vi "sweep_gate_read_lockin.vi"() -> ()   [LabVIEW 2024]
uses:
  <vilib>/Analysis/1siggen.llb/Ramp Pattern by Delta.vi
  <vilib>/Utility/file.llb/Write Delimited Spreadsheet (string).vi
  <vilib>/Utility/file.llb/Write Delimited Spreadsheet (DBL).vi
  C:/Users/Public/OneDrive/Desktop/Keithley_2450_2470_1_4_0_LV2015_NewReadme2_2450-LV2015-1.4.0/Keithley 2450/Keithley 2450.lvlib
  <vilib>/Analysis/NI_AALBase.lvlib
panel:
  in  "Wait for Current Meas":u32=100
  in  "Number of Current Meas":u32=100
  out "Actual voltage":dbl
  in  "Loop?":bool=TRUE
  out "Current set voltage":dbl
  in  "V stepsize":dbl
  in  "start V":dbl
  in  "End V":dbl
  in  "Wait for lock in meas (ms)":i32=2000
  in  "File Path":path=path "C:/Users/Public/OneDrive/Desktop/test.txt"
  out "错误输出":errorcluster
  out "Channel AWaveform Chart":dbl[](graph)
  in  "Channel A Waveform Display":string(combo)="A-R"
  in  "Channel B Waveform Display":string(combo)="Channel_B_Rh1"
  out "Channel B Waveform Chart":dbl[](graph)
  out "AUX-ADC4 (V)":sgl format="%.3f"
  out "AUX-ADC3 (V)":sgl format="%.3f"
  out "AUX-ADC1 (V)":sgl format="%.3f"
  out "AUX-ADC2 (V)":sgl format="%.3f"
  out "R":sgl caption="R (Vrms)" format="%.3p"
  out "X":sgl caption="X (Vrms)" format="%.3p"
  out "Y":sgl caption="Y (Vrms)" format="%.3p"
  out "θ (°)":sgl caption="θ (deg)" format="%.2f"
  out "频率 (Hz)":sgl caption="Freq (Hz)" format="%#.3f"
  out "噪声":sgl caption="Noise(Vrms)" format="%.3p"
  out "Rh1":sgl caption="Rh1 (Vrms)" format="%.3p"
  out "θh1 (°)":sgl caption="θh1 (deg)" format="%.2f"
  out "Xh1":sgl caption="Xh1 (Vrms)" format="%.3p"
  out "Yh1":sgl caption="Yh1 (Vrms)" format="%.3p"
  out "X 2":sgl caption="X (Vrms)" format="%.3p"
  out "Y 2":sgl caption="Y (Vrms)" format="%.3p"
  out "R 2":sgl caption="R (Vrms)" format="%.3p"
  out "θ (°) 2":sgl caption="θ (deg)" format="%.2f"
  out "频率 (Hz) 2":sgl caption="Freq (Hz)" format="%#.3f"
  out "噪声 2":sgl caption="Noise(Vrms)" format="%.3p"
  out "Xh1 2":sgl caption="Xh1 (Vrms)" format="%.3p"
  out "Yh1 2":sgl caption="Yh1 (Vrms)" format="%.3p"
  out "Rh1 2":sgl caption="Rh1 (Vrms)" format="%.3p"
  out "θh1 (°) 2":sgl caption="θh1 (deg)" format="%.2f"
  in  "A Sensitivity":u16(ring)=20 items=["1 nV/fA", "2 nV/fA", "5 nV/fA", "10 nV/fA", "20 nV/fA", "50 nV/fA", "100 nV/fA", "200 nV/fA", "500 nV/fA", "1 uV/pA", "2 uV/pA", "5 uV/pA", "10 uV/pA", "20 uV/pA", "50 uV/pA", "100 uV/pA", "200 uV/pA", "500 uV/pA", "1 mV/nA", "2 mV/nA", "5 mV/nA", "10 mV/nA", "20 mV/nA", "50 mV/nA", "100 mV/nA", "200 mV/nA", "500 mV/nA", "1 V/uA"]
  in  "B Sensitivity":u16(ring)=17 items=["1 nV/fA", "2 nV/fA", "5 nV/fA", "10 nV/fA", "20 nV/fA", "50 nV/fA", "100 nV/fA", "200 nV/fA", "500 nV/fA", "1 uV/pA", "2 uV/pA", "5 uV/pA", "10 uV/pA", "20 uV/pA", "50 uV/pA", "100 uV/pA", "200 uV/pA", "500 uV/pA", "1 mV/nA", "2 mV/nA", "5 mV/nA", "10 mV/nA", "20 mV/nA", "50 mV/nA", "100 mV/nA", "200 mV/nA", "500 mV/nA", "1 V/uA"]
  out "序列号":string
  in  "Num Lock in Points":i32=100
  in  "OE1022D":refnum<visa-resource-name>="COM6"
  in  "Limit Reached 2":bool
  in  "Current Compliance Limit (0.1)":dbl=5e-08
  in  "Time between Current Meas (ms)":u32=100
  out "Current":dbl caption="Measured Current (A)"
  out "XY Graph":cluster{dbl[], dbl[]}(graph)
  out "error out":errorcluster
  in  "error in (no error)":errorcluster
  in  "VISA resource name 2":refnum<visa-resource-name>="GPIB0::18::INSTR"
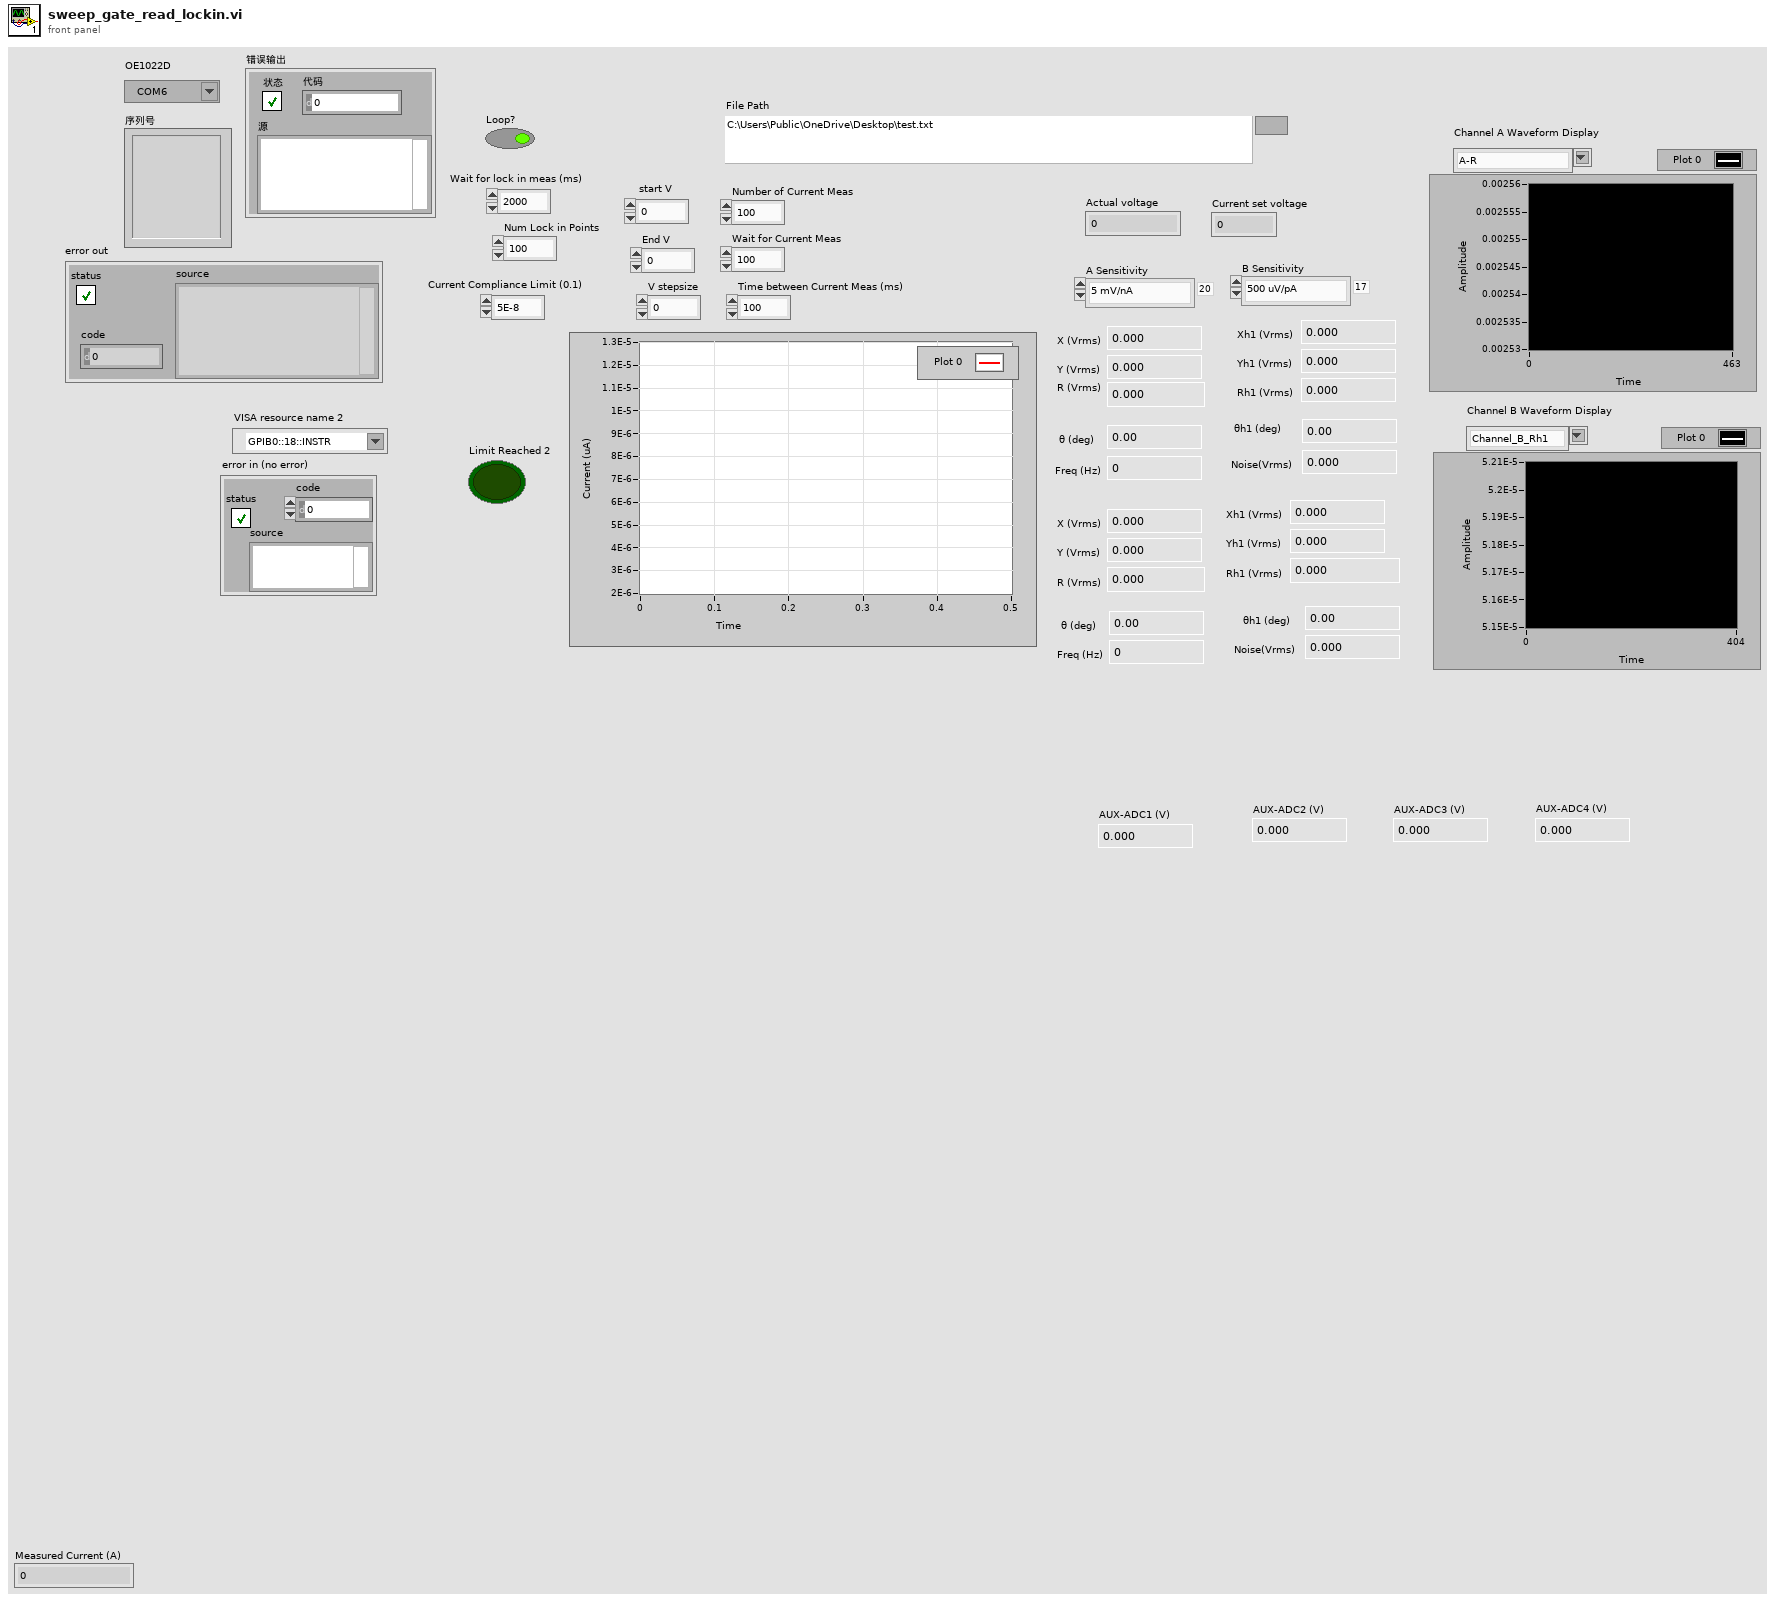
[diagram p1: front panel]
types:
  T1 = cluster{"AD1":dbl[], "AD2":dbl[], "AD3":dbl[], "AD4":dbl[]}
  T2 = cluster{"XB":dbl[], "YB":dbl[], "FrequencyB":dbl[], "NoiseB":dbl[], "Xh1B":dbl[], "Yh1B":dbl[], "Xh2B":dbl[], "Yh2B":dbl[], "Xh2B":dbl[]}
  T3 = cluster{"XA":dbl[], "YA":dbl[], "FrequencyA":dbl[], "NoiseA":dbl[], "Xh1A":dbl[], "Yh1A":dbl[], "Xh2A":dbl[], "Yh2A":dbl[]}
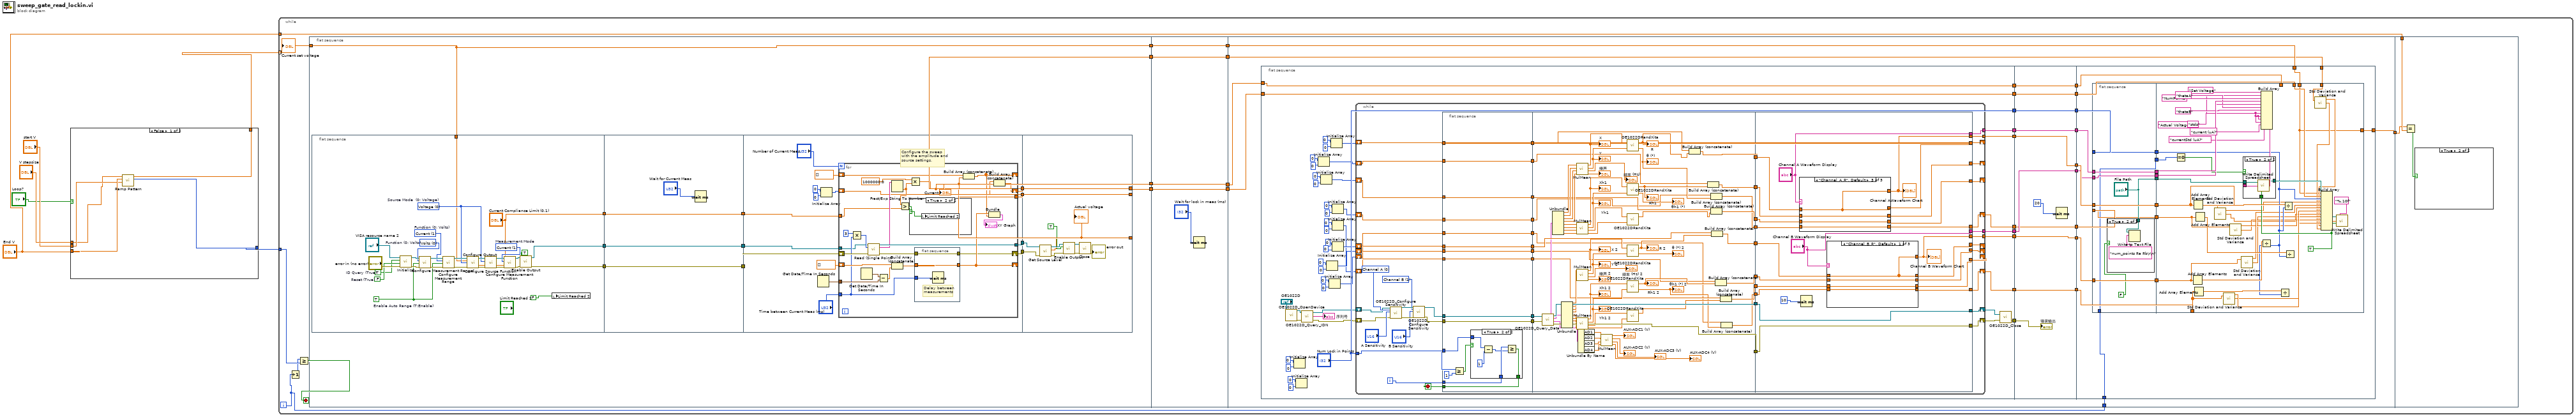
[diagram p0: block diagram]
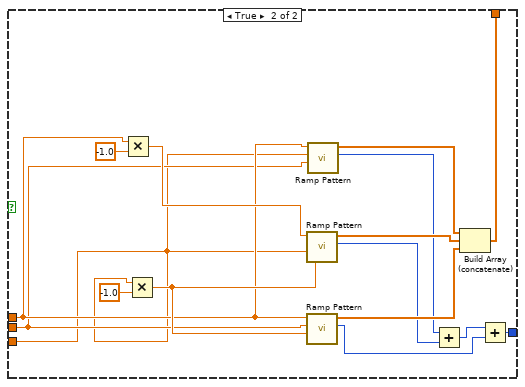
[diagram p2: hidden frame]
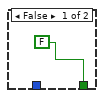
[diagram p4: hidden frame]
diagram:
  n1 = case shown="False" "Loop?" {
    tunnel: [w8 w20] -> w6
    tunnel: [w7 w15] -> w5
    tunnel: "V stepsize" -> [w9 w14]
    tunnel: "start V" -> [w10 w13]
    tunnel: "End V" -> [w11 w12]
    frame False {
      n2 = call-poly <vilib>:"Ramp Pattern.vi"("start"=w10, "end"=w11, "delta"=w9) -> ("samples"=w7:i32, "Ramp Pattern"=w8:dbl[])  [unwired: 6 in, 1 out]
    }
    frame True {
      n3 = Multiply(x=w14, y=-1.0) -> (x*y=w25:dbl)
      n4 = Multiply(x=w12, y=-1.0) -> (x*y=w24:dbl)
      n5 = call-poly <vilib>:"Ramp Pattern.vi"("start"=w12, "end"=w24, "delta"=w25) -> ("samples"=w18:i32, "Ramp Pattern"=w22:dbl[])  [unwired: 6 in, 1 out]
      n6 = call-poly <vilib>:"Ramp Pattern.vi"("start"=w24, "end"=w13, "delta"=w14) -> ("samples"=w17:i32, "Ramp Pattern"=w21:dbl[])  [unwired: 6 in, 1 out]
      n7 = call-poly <vilib>:"Ramp Pattern.vi"("start"=w13, "end"=w12, "delta"=w14) -> ("samples"=w19:i32, "Ramp Pattern"=w23:dbl[])  [unwired: 6 in, 1 out]
      n8 = Add(x=w19, y=w18) -> (x+y=w16:i32)
      n9 = Build Array (concatenate)(w23, w22, w21) -> (w20:dbl[])
      n10 = Add(x=w16, y=w17) -> (x+y=w15:i32)
    }
  }
  n11 = while {
    tunnel: w6 -> [w40] mode=indexing
    tunnel: w5 -> [w42]
    tunnel: "End V" -> [w28]
    i -> [w30]
    stop <- w41 stop-if-true
    n12 = Increment(x=w30) -> (x+1=w39:i32)
    n13 = Greater Or Equal?(x=w39, y=w42) -> (x >= y?=w41:bool)
    n14 = flat-sequence {
      tunnel: w40 -> [w49]
      tunnel: [w56] -> w37
      tunnel: [w49] -> w36
      tunnel: [w50] -> w33
      tunnel: [w55] -> w31
      tunnel: [w146] -> w38
      tunnel: w37 -> [w146]
      tunnel: w36 -> [w145]
      tunnel: [w145] -> w35
      tunnel: [w144] -> w34
      tunnel: w33 -> [w144]
      tunnel: [w143] -> w32
      tunnel: w31 -> [w143]
      tunnel: w38 -> [w157]
      tunnel: w35 -> [w154]
      tunnel: w34 -> [w153]
      tunnel: w32 -> [w150]
      tunnel: w30 -> [w149]
      tunnel: [w148] -> w29
      tunnel: w29 -> [w504]
      tunnel: w28 -> [w505]
      frame #0 {
        n15 = flat-sequence {
          tunnel: w49 -> [w60]
          tunnel: [w59] -> w48
          tunnel: ["Current Compliance Limit (0.1)"] -> w46
          tunnel: [w57] -> w44
          tunnel: w48 -> [w87]
          tunnel: [w87] -> w47
          tunnel: w46 -> [w86]
          tunnel: [w86] -> w45
          tunnel: w44 -> [w85]
          tunnel: [w85] -> w43
          tunnel: [w98] -> w54
          tunnel: [w97] -> w53
          tunnel: [w93] -> w52
          tunnel: [w92] -> w51
          tunnel: w47 -> [w90]
          tunnel: w45 -> [w89]
          tunnel: w43 -> [w88]
          tunnel: [w141] -> w55
          tunnel: [w142] -> w56
          tunnel: w54 -> [w134]
          tunnel: w53 -> [w135]
          tunnel: w52 -> [w142]
          tunnel: w51 -> [w141]
          tunnel: [w132] -> w50
          frame #0 {
            w61 = u16 0 items=["Voltage", "Current"]  # Source Mode  (0: Voltage)
            w62 = u16 1 items=["Volts", "Current", "Auto Resistance", "Manual Resistance", "Digitize Voltage", "Digitize Current"]  # Measurement Mode
            w66 = TRUE  # Enable Auto Range (T:Enable)
            w64 = u16 1 items=["Volts", "Current", "Resistance"]  # Function (0: Volts)
            w65 = u16 0 items=["Volts", "Current", "Resistance"]  # Function (0: Volts)
            w68 = FALSE  # Reset (True)
            w67 = TRUE  # ID Query (True)
            n16 = call "Initialize.vi"("error in (no error)"="error in (no error)", "Reset (True)"=w68, "ID Query (True)"=w67, "VISA resource name"="VISA resource name 2") -> ("error out"=w72:errorcluster, "VISA resource name out"=w71:refnum<visa-resource-name>)  [unwired: 6 in]
            n17 = call "Configure Measurement Range.vi"("error in (no error)"=w72, "Enable Auto Range (T:Enable)"=w66, "Function (0: Volts)"=w65, "VISA resource name"=w71) -> ("error out"=w70:errorcluster, "VISA resource name out"=w69:refnum<visa-resource-name>)  [unwired: 6 in]
            n18 = call "Configure Measurement Range.vi"("error in (no error)"=w70, "Enable Auto Range (T:Enable)"=w66, "Function (0: Volts)"=w64, "VISA resource name"=w69) -> ("error out"=w80:errorcluster, "VISA resource name out"=w81:refnum<visa-resource-name>)  [unwired: 6 in]
            n19 = call "Configure Output.vi"("VISA resource name"=w81, "Source Level (0)"=w60, "Source Mode  (0: Voltage)"=w61, "Source Limit Level (0.1)"="Current Compliance Limit (0.1)", "error in (no error)"=w80) -> ("VISA resource name out"=w73:refnum<visa-resource-name>, "error out"=w74:errorcluster)  [unwired: 9 in]
            n20 = call "Configure Source Function.vi"("error in (no error)"=w74, "Function (0: Volts)"=w61, "VISA resource name"=w73) -> ("error out"=w76:errorcluster, "VISA resource name out"=w77:refnum<visa-resource-name>)  [unwired: 7 in]
            n21 = call "Configure Measurement Function.vi"("error in (no error)"=w76, "Function (0: Volts)"=w62, "VISA resource name"=w77) -> ("error out"=w78:errorcluster, "VISA resource name out"=w79:refnum<visa-resource-name>)  [unwired: 7 in]
            n22 = call "Enable Output.vi"("error in (no error)"=w78, "Enable Output (T: Enable)"=TRUE, "VISA resource name"=w79) -> ("error out"=w57:errorcluster, "VISA resource name out"=w59:refnum<visa-resource-name>)  [unwired: 7 in]
            n23 = local write "Limit Reached 2"(FALSE) -> ()
          }
          frame #1 {
            n24 = Wait (ms)(milliseconds to wait="Wait for Current Meas") -> ()  [unwired: 1 out]
          }
          frame #2 {
            # "Configure the sweep with the amplitude and source settings."
            n25 = Get Date/Time In Seconds() -> (seconds since 1Jan1904=w102:timestamp)
            n26 = Initialize Array(0, 0) -> (w94:i32[])
            n27 = for {
              N: "Number of Current Meas" -> [_]
              shift-right: [w116] -> w97
              shift-left: w88 -> [w118]
              tunnel: w102 -> [w126]
              shift-right: [w122] -> _
              shift-left: dbl[] [] -> [w125]
              shift-right: [w121] -> _
              shift-left: dbl[] [] -> [w124]
              tunnel: "Time between Current Meas (ms)" -> [w114]
              tunnel: [w112] -> w98
              tunnel: w89 -> [w110]
              tunnel: [w106] -> w93
              shift-right: [w108] -> w92
              shift-left: w94 -> [w107]
              tunnel: w90 -> [w104]
              n28 = Multiply(x=u32 3, y=w114) -> (x*y=w115:u32)
              n29 = Get Date/Time In Seconds() -> (seconds since 1Jan1904=w127:timestamp)
              n30 = call "Read (Single Point).vi"("VISA resource name"=w104, "Timeout (10000 ms)"=w115, "error in (no error)"=w118) -> ("VISA resource name out"=w112:refnum<visa-resource-name>, "Data out"=w111:string, "error out"=w117:errorcluster)  [unwired: 10 in]
              n31 = Subtract(x=w127, y=w126) -> (x-y=w119:dbl)
              n32 = Fract/Exp String To Number(string=w111) -> (number=w103:dbl)  [unwired: 3 in, 1 out]
              n33 = Build Array (concatenate)(w125, w119) -> (w123:dbl[])
              n34 = Greater?(x=w103, y=w110) -> (0:w109:bool)
              n35 = case shown="True" w109 {
                selector: w109 -> [_ w128]
                frame False {
                }
                frame True {
                  n36 = local write "Limit Reached 2"(w128) -> ()
                }
              }
              n37 = Multiply(x=1000000.0, y=w103) -> (x*y=w106:dbl)
              "Current" <- w106
              n38 = flat-sequence {
                tunnel: w123 -> [w131]
                tunnel: [w131] -> w122
                tunnel: w114 -> [w130]
                tunnel: w117 -> [w129]
                tunnel: [w129] -> w116
                frame #0 {
                  # "Delay between\nmeasurements"
                  n39 = Wait (ms)(milliseconds to wait=w130) -> ()  [unwired: 1 out]
                }
              }
              n40 = Build Array (concatenate)(w124, w106) -> (w121:dbl[])
              n41 = Bundle(w122, w121) -> (→"XY Graph":cluster{dbl[], dbl[]})  [unwired: 1 in]
              n42 = Build Array (concatenate)(w107, w106) -> (w108:dbl[])
            }
          }
          frame #3 {
            n43 = call "Get Source Level.vi"("error in (no error)"=w135, "VISA resource name"=w134) -> ("error out"=w139:errorcluster, "Voltage Level Out"=w132:dbl, "VISA resource name out"=w140:refnum<visa-resource-name>)  [unwired: 6 in, 1 out]
            "Actual voltage" <- w132
            n44 = call "Enable Output.vi"("error in (no error)"=w139, "Enable Output (T: Enable)"=TRUE, "VISA resource name"=w140) -> ("error out"=w137:errorcluster, "VISA resource name out"=w136:refnum<visa-resource-name>)  [unwired: 7 in]
            n45 = call "Close.vi"("error in (no error)"=w137, "VISA resource name"=w136) -> ("error out"=→"error out":errorcluster)  [unwired: 9 in]
          }
        }
      }
      frame #1 {
        n46 = Wait (ms)(milliseconds to wait="Wait for lock in meas (ms)") -> ()  [unwired: 1 out]
      }
      frame #2 {
        n47 = flat-sequence {
          tunnel: [w195] -> w172
          tunnel: [w194] -> w171
          tunnel: ["Num Lock in Points"] -> w170
          tunnel: [w189] -> w169
          tunnel: [w193] -> w168
          tunnel: [w192] -> w167
          tunnel: [w179] -> w166
          tunnel: [w180] -> w165
          tunnel: w157 -> [w174]
          tunnel: [w174] -> w155
          tunnel: w153 -> [w173]
          tunnel: [w173] -> w151
          tunnel: w172 -> [w425]
          tunnel: [w425] -> w164
          tunnel: w171 -> [w424]
          tunnel: [w424] -> w163
          tunnel: w170 -> [w423]
          tunnel: [w423] -> w162
          tunnel: w169 -> [w421]
          tunnel: [w420] -> w161
          tunnel: w168 -> [w420]
          tunnel: w167 -> [w419]
          tunnel: [w419] -> w160
          tunnel: [w418] -> w159
          tunnel: w166 -> [w418]
          tunnel: w165 -> [w417]
          tunnel: [w417] -> w158
          tunnel: [w416] -> w156
          tunnel: w155 -> [w416]
          tunnel: [w415] -> w152
          tunnel: w151 -> [w415]
          tunnel: w164 -> [w442]
          tunnel: w163 -> [w441]
          tunnel: w162 -> [w440]
          tunnel: w161 -> [w438]
          tunnel: w160 -> [w437]
          tunnel: w159 -> [w435]
          tunnel: w158 -> [w433]
          tunnel: w156 -> [w432]
          tunnel: w154 -> [w431]
          tunnel: w152 -> [w430]
          tunnel: w150 -> [w429]
          tunnel: w149 -> [w427]
          tunnel: [w426] -> w148
          frame #0 {
            n48 = call "OE1022D_OpenDevice.vi"("VISA resource name"="OE1022D") -> ("VISA资源名称输出"=w217:refnum<visa-resource-name>, "错误输出"=w216:errorcluster)  [unwired: 17 in]
            n49 = Initialize Array(0, 0) -> ()  [unwired: 1 out]
            n50 = Initialize Array(0, 0) -> ()  [unwired: 1 out]
            n51 = call "OE1022D_Query_IDN.vi"("错误输入（无错误）"=w216, "VISA resource name"=w217) -> ("错误输出"=w187:errorcluster, "序列号"=→"序列号":string, "VISA resource name out"=w188:refnum<visa-resource-name>)  [unwired: 1 in]
            n52 = Initialize Array(0, 0) -> (w202:i32[])
            n53 = Initialize Array(0, 0) -> (w203:i32[])
            n54 = Initialize Array(0, 0) -> (w196:i32[])
            n55 = Initialize Array(0, 0) -> (w197:i32[])
            n56 = Initialize Array(0, 0) -> (w213:i32[])
            n57 = Initialize Array(0, 0) -> (w181:i32[])
            n58 = Initialize Array(0, 0) -> (w208:i32[])
            n59 = Initialize Array(0, 0) -> (w182:i32[])
            n60 = while {
              shift-right: [w270] -> _
              shift-left: w213 -> [w269]
              shift-right: [w267] -> _
              shift-left: w208 -> [w266]
              tunnel: "Num Lock in Points" -> [w259]
              shift-right: [w247] -> _
              shift-left: w202 -> [w249]
              shift-right: [w243] -> _
              shift-left: w203 -> [w246]
              shift-right: [w236] -> _
              shift-left: w196 -> [w242]
              shift-right: [w235] -> _
              shift-left: w197 -> [w241]
              tunnel: [w234] -> w195
              tunnel: [w233] -> w194
              tunnel: [w232] -> w193
              tunnel: [w231] -> w192
              shift-right: [w230] -> w191
              shift-left: w187 -> [w227]
              shift-right: [w229] -> w190
              shift-left: w188 -> [w228]
              shift-right: [w219] -> w179
              shift-left: w182 -> [w223]
              shift-right: [w220] -> w180
              shift-left: w181 -> [w221]
              i -> [w261]
              stop <- w260 stop-if-true
              w252 = u8 1 items=["Channel A", "Channel B"] ("OE1022D A/B")
              w258 = u8 0 items=["Channel A", "Channel B"] ("OE1022D A/B")
              n61 = call "OE1022D_Configure Sensitivity.vi"("VISA resource name"=w228, "OE1022D A/B"=w258, "Sensitivity"="A Sensitivity", "error in (no error)"=w227) -> ("VISA resource name out"=w253:refnum<visa-resource-name>, "error out"=w254:errorcluster)  [unwired: 14 in]
              n62 = call "OE1022D_Configure Sensitivity.vi"("VISA resource name"=w253, "OE1022D A/B"=w252, "Sensitivity"="B Sensitivity", "error in (no error)"=w254) -> ("VISA resource name out"=w256:refnum<visa-resource-name>, "error out"=w255:errorcluster)  [unwired: 14 in]
              n63 = flat-sequence {
                tunnel: w266 -> [w285]
                tunnel: w269 -> [w286]
                tunnel: w256 -> [w287]
                tunnel: w255 -> [w288]
                tunnel: [w288] -> w265
                tunnel: [w287] -> w264
                tunnel: [w286] -> w263
                tunnel: [w285] -> w262
                tunnel: w261 -> [w284]
                tunnel: [w283] -> w260
                tunnel: w259 -> [w281]
                tunnel: [w279] -> w250
                tunnel: w249 -> [w279]
                tunnel: w246 -> [w278]
                tunnel: [w278] -> w245
                tunnel: w242 -> [w277]
                tunnel: w241 -> [w276]
                tunnel: [w277] -> w240
                tunnel: [w276] -> w239
                tunnel: [w275] -> w224
                tunnel: w223 -> [w275]
                tunnel: [w274] -> w222
                tunnel: w221 -> [w274]
                tunnel: [w365] -> w273
                tunnel: [w364] -> w272
                tunnel: [w317] -> w271
                tunnel: [w313] -> w268
                tunnel: w265 -> [w367]
                tunnel: w264 -> [w366]
                tunnel: w263 -> [w318]
                tunnel: w262 -> [w315]
                tunnel: w250 -> [w311]
                tunnel: [w310] -> w248
                tunnel: w245 -> [w308]
                tunnel: [w307] -> w244
                tunnel: w240 -> [w303]
                tunnel: w239 -> [w304]
                tunnel: [w302] -> w238
                tunnel: [w301] -> w237
                tunnel: [w297] -> w226
                tunnel: [w299] -> w225
                tunnel: w224 -> [w296]
                tunnel: w222 -> [w295]
                tunnel: w273 -> [w388]
                tunnel: w272 -> [w389]
                tunnel: w271 -> [w387]
                tunnel: [w385] -> w270
                tunnel: w268 -> [w381]
                tunnel: [w380] -> w267
                tunnel: [w389] -> w229
                tunnel: [w388] -> w230
                tunnel: w248 -> [w386]
                tunnel: [w384] -> w247
                tunnel: w244 -> [w383]
                tunnel: [w382] -> w243
                tunnel: w238 -> [w376]
                tunnel: w237 -> [w379]
                tunnel: [w378] -> w236
                tunnel: [w377] -> w235
                tunnel: [w375] -> w234
                tunnel: [w374] -> w233
                tunnel: ["Channel A Waveform Display"] -> w232
                tunnel: ["Channel B Waveform Display"] -> w231
                tunnel: w226 -> [w370]
                tunnel: [w369] -> w219
                tunnel: [w368] -> w220
                tunnel: w225 -> [w371]
                frame #0 {
                  n64 = Greater Or Equal?(x=w281, y=1) -> (x >= y?=w280:bool)
                  n65 = case shown="True" w280 {
                    tunnel: w284 -> [_ w294]
                    tunnel: [FALSE w293] -> w283
                    tunnel: w281 -> [_ w290]
                    frame False {
                    }
                    frame True {
                      n66 = Subtract(x=w290, y=1) -> (x-y=w291:i32)
                      n67 = Greater Or Equal?(x=w294, y=w291) -> (x >= y?=w293:bool)
                    }
                  }
                }
                frame #1 {
                  n68 = call "OE1022D_Query_Data.vi"("错误输入（无错误）"=w367, "VISA resource name"=w366) -> ("error out"=w365:errorcluster, "输出簇ADC"=w321:T1, "输出簇B"=w320:T2, "VISA resource name out"=w364:refnum<visa-resource-name>, "输出簇A"=w314:T3)  [unwired: 3 in]
                  n69 = Unbundle(w314) -> ("XA"=w326:dbl[], "YA"=w327:dbl[], "FrequencyA"=w328:dbl[], "NoiseA"=w329:dbl[], "Xh1A"=w334:dbl[], "Yh1A"=w335:dbl[], "Xh2A"=w336:dbl[], "Yh2A"=w337:dbl[])
                  n70 = Unbundle(w320) -> ("XB"=w350:dbl[], "YB"=w349:dbl[], "FrequencyB"=w348:dbl[], "NoiseB"=w347:dbl[], "Xh1B"=w346:dbl[], "Yh1B"=w345:dbl[], "Xh2B"=w344:dbl[], "Yh2B"=w343:dbl[])  [unwired: 1 out]
                  n71 = call "MulMean.vi"("IN 4"=w329, "IN 3"=w328, "IN 2"=w327, "IN 1"=w326) -> ("mean 4"=→"噪声":dbl, "mean 3"=→"频率 (Hz)":dbl, "mean 2"=w332:dbl, "mean 1"=w331:dbl)  [unwired: 4 in]
                  "X" <- w331
                  "Y" <- w332
                  n72 = call "MulMean.vi"("IN 4"=w337, "IN 3"=w336, "IN 2"=w335, "IN 1"=w334) -> ("mean 4"=w342:dbl, "mean 3"=w341:dbl, "mean 2"=w339:dbl, "mean 1"=w338:dbl)  [unwired: 4 in]
                  "Xh1" <- w338
                  "Yh1" <- w339
                  n73 = call "MulMean.vi"("IN 4"=w347, "IN 3"=w348, "IN 2"=w349, "IN 1"=w350) -> ("mean 4"=→"噪声 2":dbl, "mean 3"=→"频率 (Hz) 2":dbl, "mean 2"=w355:dbl, "mean 1"=w354:dbl)  [unwired: 4 in]
                  "X 2" <- w354
                  "Y 2" <- w355
                  n74 = call "MulMean.vi"("IN 4"=w343, "IN 3"=w344, "IN 2"=w345, "IN 1"=w346) -> ("mean 4"=w359:dbl, "mean 3"=w358:dbl, "mean 2"=w357:dbl, "mean 1"=w356:dbl)  [unwired: 4 in]
                  "Xh1 2" <- w356
                  "Yh1 2" <- w357
                  n75 = Unbundle By Name(w321) -> ("AD1"=w360:dbl[], "AD2"=w361:dbl[], "AD3"=w362:dbl[], "AD4"=w363:dbl[])
                  n76 = call "MulMean.vi"("IN 4"=w363, "IN 3"=w362, "IN 2"=w361, "IN 1"=w360) -> ("mean 4"=→"AUX-ADC4 (V)":dbl, "mean 3"=→"AUX-ADC3 (V)":dbl, "mean 2"=→"AUX-ADC2 (V)":dbl, "mean 1"=→"AUX-ADC1 (V)":dbl)  [unwired: 4 in]
                  n77 = call "OE1022DRandXita.vi"("Y"=w332, "X"=w331) -> ("θ (°)"=w298:dbl, "R"=w319:dbl)
                  "R" <- w319
                  "θ (°)" <- w298
                  n78 = call "OE1022DRandXita.vi"("Y"=w339, "X"=w338) -> ("θ (°)"=→"θh1 (°)":dbl, "R"=w312:dbl)
                  "Rh1" <- w312
                  n79 = call "OE1022DRandXita.vi"("Y"=w342, "X"=w341) -> ("R"=w309:dbl)  [unwired: 1 out]
                  n80 = call "OE1022DRandXita.vi"("Y"=w355, "X"=w354) -> ("θ (°)"=→"θ (°) 2":dbl, "R"=w316:dbl)
                  "R 2" <- w316
                  n81 = call "OE1022DRandXita.vi"("Y"=w357, "X"=w356) -> ("θ (°)"=w300:dbl, "R"=w306:dbl)
                  "Rh1 2" <- w306
                  "θh1 (°) 2" <- w300
                  n82 = call "OE1022DRandXita.vi"("Y"=w359, "X"=w358) -> ("R"=w305:dbl)  [unwired: 1 out]
                  n83 = Build Array (concatenate)(w318, w319) -> (w317:dbl[])
                  n84 = Build Array (concatenate)(w311, w312) -> (w310:dbl[])
                  n85 = Build Array (concatenate)(w296, w298) -> (w297:dbl[])
                  n86 = Build Array (concatenate)(w308, w309) -> (w307:dbl[])
                  n87 = Build Array (concatenate)(w315, w316) -> (w313:dbl[])
                  n88 = Build Array (concatenate)(w303, w306) -> (w302:dbl[])
                  n89 = Build Array (concatenate)(w304, w305) -> (w301:dbl[])
                  n90 = Build Array (concatenate)(w295, w300) -> (w299:dbl[])
                }
                frame #2 {
                  n91 = case shown="\"Channel_A_R\", Default" "Channel A Waveform Display" {
                    tunnel: w387 -> [w406 w410 w412]
                    tunnel: [w406 w410 w412] -> w385
                    tunnel: w386 -> [w404 w409 w414]
                    tunnel: [w404 w409 w414] -> w384
                    tunnel: w383 -> [w405 w408 w413]
                    tunnel: [w405 w408 w413] -> w382
                    tunnel: [w404 w408 w412] -> w375
                    tunnel: w370 -> [w403 w407 w411]
                    tunnel: [w403 w407 w411] -> w369
                    frame "Channel_A_Rh1" {
                    }
                    frame "Channel_A_Rh2" {
                    }
                    frame "Channel_A_R", Default {
                    }
                  }
                  "Channel AWaveform Chart" <- w375
                  n92 = Wait (ms)(milliseconds to wait=10) -> ()  [unwired: 1 out]
                  n93 = case shown="\"Channel_B_R\", Default" "Channel B Waveform Display" {
                    tunnel: [w394 w396 w400] -> w374
                    tunnel: w381 -> [w394 w398 w402]
                    tunnel: [w394 w398 w402] -> w380
                    tunnel: w379 -> [w393 w397 w400]
                    tunnel: [w393 w397 w400] -> w377
                    tunnel: [w392 w396 w401] -> w378
                    tunnel: w376 -> [w392 w396 w401]
                    tunnel: w371 -> [w391 w395 w399]
                    tunnel: [w391 w395 w399] -> w368
                    frame "Channel_B_R", Default {
                    }
                    frame "Channel_B_Rh1" {
                    }
                    frame "Channel_B_Rh2" {
                    }
                  }
                  "Channel B Waveform Chart" <- w374
                }
              }
            }
            n94 = call "OE1022D_Close.vi"("错误输入（无错误）"=w191, "VISA resource name"=w190) -> ("错误输出"=w189:errorcluster)  [unwired: 1 in]
          }
          frame #1 {
            n95 = Wait (ms)(milliseconds to wait=20) -> ()  [unwired: 1 out]
            "错误输出" <- w421
          }
          frame #2 {
            n96 = flat-sequence {
              tunnel: w440 -> [w453]
              tunnel: w441 -> [w454]
              tunnel: w442 -> [w455]
              tunnel: [w455] -> w446
              tunnel: [w454] -> w445
              tunnel: [w453] -> w444
              tunnel: ["File Path"] -> w443
              tunnel: [w450] -> w439
              tunnel: w438 -> [w450]
              tunnel: w437 -> [w449]
              tunnel: [w449] -> w436
              tunnel: w435 -> [w448]
              tunnel: [w448] -> w434
              tunnel: [w447] -> w428
              tunnel: w427 -> [w447]
              tunnel: w446 -> [w478]
              tunnel: w445 -> [w481]
              tunnel: w444 -> [w484]
              tunnel: w443 -> [w492]
              tunnel: w439 -> [w490]
              tunnel: w436 -> [w489]
              tunnel: w434 -> [w479]
              tunnel: w433 -> [w480]
              tunnel: w432 -> [_]
              tunnel: w431 -> [w458]
              tunnel: w430 -> [w465]
              tunnel: w429 -> [w463]
              tunnel: w428 -> [w460]
              tunnel: [w458] -> w426
              frame #0 {
                n97 = case shown="True" FALSE {
                  tunnel: "File Path" -> [_ w457]
                  frame False {
                  }
                  frame True {
                    n98 = Write to Text File(file (use dialog)=w457, text="num_points Ra Rb\r\n") -> ()  [unwired: 2 in, 3 out]
                  }
                }
              }
              frame #1 {
                w469 = "stds"
                w491 = TRUE
                n99 = Equal To 0?(x=w460) -> (x = 0?=w459:bool)
                n100 = Add Array Elements(numeric array=w481) -> (sum=w494:dbl)
                n101 = Add Array Elements(numeric array=w478) -> (sum=w496:dbl)
                n102 = Add Array Elements(numeric array=w480) -> (sum=w485:dbl)
                n103 = Add Array Elements(numeric array=w479) -> (sum=w486:dbl)
                n104 = call <vilib>:"Std Deviation and Variance.vi"("X"=w478) -> ("mean"=w477:dbl, "standard deviation"=w471:dbl)  [unwired: 1 in, 1 out]
                n105 = call <vilib>:"Std Deviation and Variance.vi"("X"=w480) -> ("mean"=w474:dbl, "standard deviation"=w473:dbl)  [unwired: 1 in, 1 out]
                n106 = call <vilib>:"Std Deviation and Variance.vi"("X"=w479) -> ("mean"=w475:dbl, "standard deviation"=w472:dbl)  [unwired: 1 in, 1 out]
                n107 = call <vilib>:"Std Deviation and Variance.vi"("X"=w481) -> ("mean"=w476:dbl, "standard deviation"=w470:dbl)  [unwired: 1 in, 1 out]
                n108 = Build Array("Set Voltage", "Actual Voltage", "NumPoints", w490, w489, "thetaA", "thetaB", w469, w469, w469, w469, "current (uA)", "currentStd (uA)") -> (w487:string[])
                n109 = case shown="True" w459 {
                  tunnel: [w498 w502] -> w493
                  tunnel: w492 -> [w498 w501]
                  tunnel: w491 -> [_ w500]
                  tunnel: w487 -> [_ w499]
                  frame False {
                  }
                  frame True {
                    n110 = call-poly <vilib>:"Write Delimited Spreadsheet.vi"("file path (dialog if empty)"=w501, "1D data"=w499, "append to file? (new file:F)"=w500) -> ("new file path (Not A Path if cancelled)"=w502:path)  [unwired: 11 in, 1 out]
                  }
                }
                n111 = Divide(x=w494, y=w484) -> ()  [unwired: 1 out]
                n112 = Divide(x=w485, y=w484) -> ()  [unwired: 1 out]
                n113 = Divide(x=w496, y=w484) -> ()  [unwired: 1 out]
                n114 = Divide(x=w486, y=w484) -> ()  [unwired: 1 out]
                n115 = call <vilib>:"Std Deviation and Variance.vi"("X"=w463) -> ("mean"=w462:dbl, "standard deviation"=w461:dbl)  [unwired: 1 in, 1 out]
                n116 = Build Array(w458, w465, w484, w477, w476, w475, w474, w471, w470, w472, w473, w462, w461) -> (w495:dbl[])
                n117 = call-poly <vilib>:"Write Delimited Spreadsheet.vi"("file path (dialog if empty)"=w493, "format (%.3f)"="%.10f", "1D data"=w495, "append to file? (new file:F)"=w491) -> ()  [unwired: 10 in, 2 out]
              }
            }
          }
        }
      }
      frame #3 {
        n118 = Equal?(x=w504, y=w505) -> (x = y?=w503:bool)
        n119 = case shown="True" w503 {
          frame False {
          }
          frame True {
          }
        }
      }
    }
    "Current set voltage" <- w40
  }
